vi "Test Motor Encoder.vi"(9 "Motor Power":i32, 10 "Encoder Setpoint":dbl format="%#_13g", 11 "Motor":i32) -> (1 "Encoder FeedBack":dbl, 2 "Done":bool, 3 "Current Motor Ref":T1={"DeviceStatus"={"status"=FALSE, "code"=0, "source"=""}, "Type"=enum."PWM", "PWM"={"Controller"=enum."Controller 1", "PWM Channel"=enum."Invalid", "DeadBand"={"Name"="", "maxPositivePwm"=0, "minPositivePwm"=0, "centerPwm"=0, "maxNegativePwm"=0, "minNegativePwm"=0, "angularRange"=0}}, "CAN"={"Device Number"=0, "Control Mode"=enum."Percent VBus", "Semaphore"=refnum, "Max Vout"=12.0, "TalonSRX Control Mode"=enum."Percent VBus"}, "Invert"=FALSE, "TransformRef"=refnum, "InvTransformRef"=refnum})   [LabVIEW 2014]
uses:
  <vilib>/Rock Robotics/WPI/MotorControl/WPI_MotorControlDeviceRef.ctl
  <vilib>/Rock Robotics/WPI/MotorControl/WPI_MotorControlType.ctl
  <vilib>/Rock Robotics/SystemInterfaces/Typedef/FPGA_TypedefDigitalModule.ctl
  <vilib>/Rock Robotics/SystemInterfaces/DIO/FPGA_DIOPWMChannel.ctl
  <vilib>/Rock Robotics/WPI/PWM/WPI_PWMDeadband.ctl
  <vilib>/Rock Robotics/WPI/CAN/Jaguar/SubVIs/WPI_CANJaguar_ControlMode.ctl
  <vilib>/Rock Robotics/WPI/CAN/TalonSRX/WPI_CANTalonSRX_APIControlMode.ctl
  <vilib>/Rock Robotics/WPI/PWM/WPI_PWMTransform_ConPane.ctl
  <vilib>/Rock Robotics/WPI/RobotDrive/WPI_RobotDriveMotorSelectorEnum.ctl
  <vilib>/Rock Robotics/WPI/RobotDrive/WPI_RobotDriveGetSetRefNum.vi
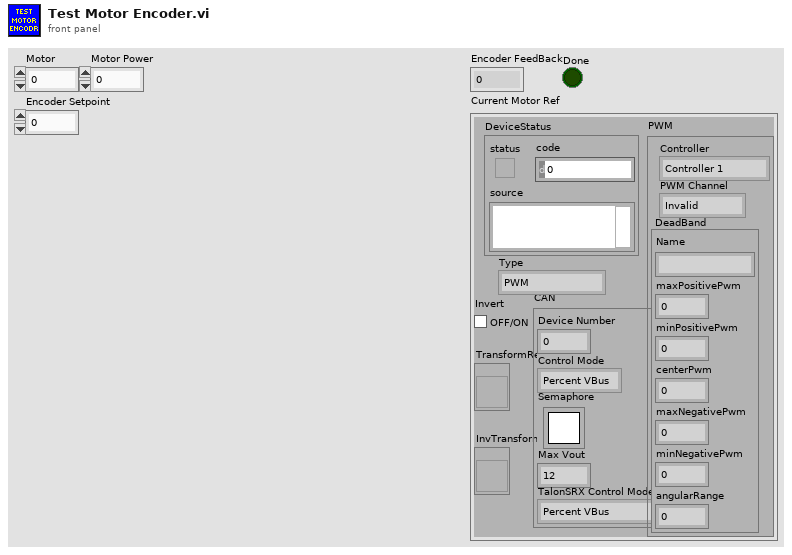
[diagram p1: front panel]
types:
  T1 = typedef "WPI_MotorControlDeviceRef.ctl" = cluster{"DeviceStatus":errorcluster, "Type":T2, "PWM":cluster{"Controller":T3, "PWM Channel":T4, "DeadBand":T5}, "CAN":cluster{"Device Number":u8, "Control Mode":T6, "Semaphore":T7, "Max Vout":dbl, "TalonSRX Control Mode":T8}, "Invert":bool, "TransformRef":T9, "InvTransformRef":T9}
  T2 = typedef "WPI_MotorControlType.ctl" = enum16{"PWM", "CAN", "CANTalonSRX"}
  T3 = typedef "FPGA_TypedefDigitalModule.ctl" = enum16{"Controller 1"}
  T4 = typedef "FPGA_DIOPWMChannel.ctl" = enum8{"PWM 0", "PWM 1", "PWM 2", "PWM 3", "PWM 4", "PWM 5", "PWM 6", "PWM 7", "PWM 8", "PWM 9", "PWM MXP 0", "PWM MXP 1", "PWM MXP 2", "PWM MXP 3", "PWM MXP 4", "PWM MXP 5", "PWM MXP 6", "PWM MXP 7", "PWM MXP 8", "PWM MXP 9", "Invalid"}
  T5 = typedef "WPI_PWMDeadband.ctl" = cluster{"Name":string, "maxPositivePwm":i32, "minPositivePwm":i32, "centerPwm":i32, "maxNegativePwm":i32, "minNegativePwm":i32, "angularRange":u16}
  T6 = typedef "WPI_CANJaguar_ControlMode.ctl" = enum8{"Percent VBus", "Current", "Speed", "Position", "Voltage"}
  T7 = typedef "Semaphore RefNum" = refnum<k1>
  T8 = typedef "WPI_CANTalonSRX_APIControlMode.ctl" = enum8{"Percent VBus", "Speed", "Position", "Slave", "Unchanged / Invalid"}
  T9 = typedef "WPI_PWMTransform_ConPane.ctl" = refnum<vi>
  T10 = typedef "WPI_RobotDriveDevRef.ctl" = cluster{"DevStatus":errorcluster, "Motors[]":T1[], "Square Inputs":bool, "Max Output":dbl}
  T11 = typedef "WPI_RobotDriveMotorSelectorEnum.ctl" = enum16{"Rear Left Motor", "Rear Right Motor", "Front Left Motor", "Front Right Motor"}
  T12 = typedef "WPI_CANTalonSRX_GlobalStatus.ctl" = cluster{"Applied Throttle":dbl, "Module Enabled":bool, "CAN Error":errorcluster, "Closed Loop Error":dbl, "Forward Limit Switch Closed":bool, "Reverse Limit Switch Closed":bool, "Sensor Position":dbl, "Sensor Velocity":dbl, "Current":dbl, "Sticky Fault - Over Temp":bool, "Sticky Fault - Under Voltage":bool, "Sticky Fault - Forward Limit":bool, "Sticky Fault - Reverse Limit":bool, "Sticky Fault - Forward Soft Limit":bool, "Sticky Fault - Reverse Soft Limit":bool, "Brake is Enabled":bool, "Encoder Position":dbl, "Encoder Velocity":dbl, "Encoder Index Count":dbl, "Encoder A Pin State":bool, "Encoder B Pin State":bool, "Encoder Index Pin State":bool, "Analog In":dbl, "Analog In Velocity":dbl, "Temperature (C)":dbl, "Battery Voltage":dbl}
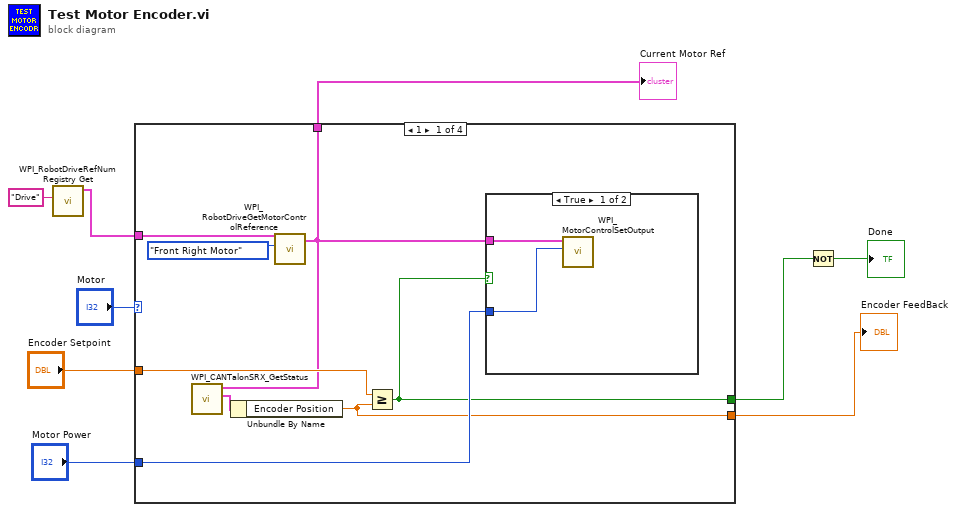
[diagram p0: block diagram]
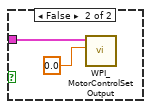
[diagram p2: hidden frame]
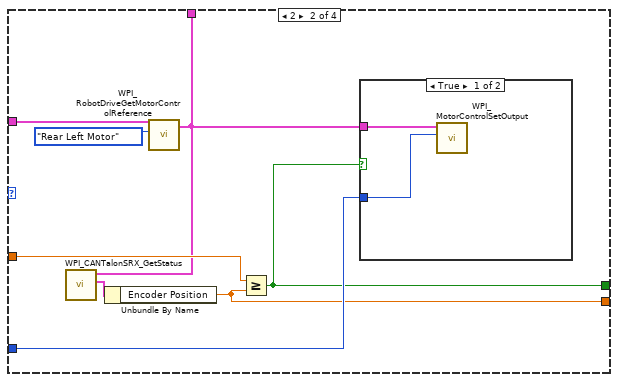
[diagram p3: hidden frame]
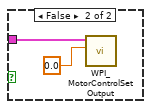
[diagram p4: hidden frame]
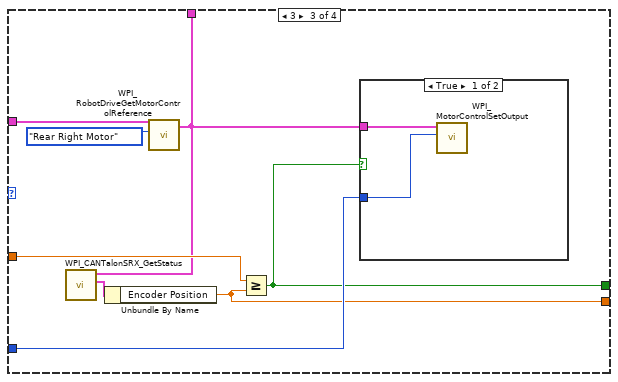
[diagram p5: hidden frame]
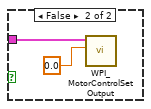
[diagram p6: hidden frame]
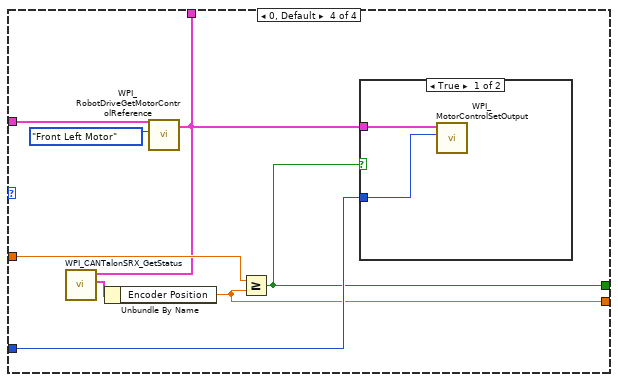
[diagram p7: hidden frame]
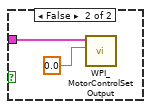
[diagram p8: hidden frame]
diagram:
  n1 = call <vilib>:"WPI_RobotDriveRefNum Registry Get.vi"("refnum name"="Drive") -> ("RobotDriveDevRef"=w7:T10)  [unwired: 9 in, 1 out]
  n2 = case shown="1" "Motor" {
    tunnel: w7 -> [w16 w28 w40 w52]
    tunnel: "Motor Power" -> [w15 w27 w39 w51]
    tunnel: "Encoder Setpoint" -> [w13 w25 w37 w49]
    tunnel: [w12 w24 w36 w48] -> w4
    tunnel: [w11 w23 w35 w47] -> w3
    tunnel: [w10 w22 w34 w46] -> w1
    frame 1 {
      n3 = call <vilib>:"WPI_RobotDriveGetMotorControlReference.vi"("MotorIndex"=WPI_RobotDriveMotorSelectorEnum."Front Right Motor", "RobotDriveDevRef"=w16) -> ("MotorControlDeviceRef"=w11:T1)  [unwired: 9 out]
      n4 = call <vilib>:"WPI_CANTalonSRX_GetStatus.vi"("CAN Talon SRX Ref"=w11) -> ("Talon SRX Status"=w14:T12)  [unwired: 8 in, 2 out]
      n5 = Unbundle By Name(w14) -> ("Encoder Position"=w12:dbl)
      n6 = Greater Or Equal?(x=w13, y=w12) -> (x >= y?=w10:bool)
      n7 = case shown="True" w10 {
        tunnel: w11 -> [w19 w21]
        tunnel: w15 -> [w18 _]
        frame True {
          n8 = call <vilib>:"WPI_MotorControlSetOutput.vi"("Output"=w18, "MotorControlDevRef"=w19) -> ()  [unwired: 7 in, 3 out]
        }
        frame False {
          n9 = call <vilib>:"WPI_MotorControlSetOutput.vi"("Output"=0.0, "MotorControlDevRef"=w21) -> ()  [unwired: 7 in, 3 out]
        }
      }
    }
    frame 2 {
      n10 = call <vilib>:"WPI_RobotDriveGetMotorControlReference.vi"("MotorIndex"=WPI_RobotDriveMotorSelectorEnum."Rear Left Motor", "RobotDriveDevRef"=w28) -> ("MotorControlDeviceRef"=w23:T1)  [unwired: 9 out]
      n11 = call <vilib>:"WPI_CANTalonSRX_GetStatus.vi"("CAN Talon SRX Ref"=w23) -> ("Talon SRX Status"=w26:T12)  [unwired: 8 in, 2 out]
      n12 = Unbundle By Name(w26) -> ("Encoder Position"=w24:dbl)
      n13 = Greater Or Equal?(x=w25, y=w24) -> (x >= y?=w22:bool)
      n14 = case shown="True" w22 {
        tunnel: w23 -> [w31 w33]
        tunnel: w27 -> [w30 _]
        frame True {
          n15 = call <vilib>:"WPI_MotorControlSetOutput.vi"("Output"=w30, "MotorControlDevRef"=w31) -> ()  [unwired: 7 in, 3 out]
        }
        frame False {
          n16 = call <vilib>:"WPI_MotorControlSetOutput.vi"("Output"=0.0, "MotorControlDevRef"=w33) -> ()  [unwired: 7 in, 3 out]
        }
      }
    }
    frame 3 {
      n17 = call <vilib>:"WPI_RobotDriveGetMotorControlReference.vi"("MotorIndex"=WPI_RobotDriveMotorSelectorEnum."Rear Right Motor", "RobotDriveDevRef"=w40) -> ("MotorControlDeviceRef"=w35:T1)  [unwired: 9 out]
      n18 = call <vilib>:"WPI_CANTalonSRX_GetStatus.vi"("CAN Talon SRX Ref"=w35) -> ("Talon SRX Status"=w38:T12)  [unwired: 8 in, 2 out]
      n19 = Unbundle By Name(w38) -> ("Encoder Position"=w36:dbl)
      n20 = Greater Or Equal?(x=w37, y=w36) -> (x >= y?=w34:bool)
      n21 = case shown="True" w34 {
        tunnel: w35 -> [w43 w45]
        tunnel: w39 -> [w42 _]
        frame True {
          n22 = call <vilib>:"WPI_MotorControlSetOutput.vi"("Output"=w42, "MotorControlDevRef"=w43) -> ()  [unwired: 7 in, 3 out]
        }
        frame False {
          n23 = call <vilib>:"WPI_MotorControlSetOutput.vi"("Output"=0.0, "MotorControlDevRef"=w45) -> ()  [unwired: 7 in, 3 out]
        }
      }
    }
    frame 0, Default {
      n24 = call <vilib>:"WPI_RobotDriveGetMotorControlReference.vi"("MotorIndex"=WPI_RobotDriveMotorSelectorEnum."Front Left Motor", "RobotDriveDevRef"=w52) -> ("MotorControlDeviceRef"=w47:T1)  [unwired: 9 out]
      n25 = call <vilib>:"WPI_CANTalonSRX_GetStatus.vi"("CAN Talon SRX Ref"=w47) -> ("Talon SRX Status"=w50:T12)  [unwired: 8 in, 2 out]
      n26 = Unbundle By Name(w50) -> ("Encoder Position"=w48:dbl)
      n27 = Greater Or Equal?(x=w49, y=w48) -> (x >= y?=w46:bool)
      n28 = case shown="True" w46 {
        tunnel: w47 -> [w55 w57]
        tunnel: w51 -> [w54 _]
        frame True {
          n29 = call <vilib>:"WPI_MotorControlSetOutput.vi"("Output"=w54, "MotorControlDevRef"=w55) -> ()  [unwired: 7 in, 3 out]
        }
        frame False {
          n30 = call <vilib>:"WPI_MotorControlSetOutput.vi"("Output"=0.0, "MotorControlDevRef"=w57) -> ()  [unwired: 7 in, 3 out]
        }
      }
    }
  }
  "Encoder FeedBack" <- w4
  "Current Motor Ref" <- w3
  n31 = Not(x=w1) -> (.not. x?=→"Done":bool)
